vi "getEnumFromName.vi"(8 "error in (no error)":errorcluster, 10 "name":string, 11 "Enumeration in":refnum<class "Enumeration.lvclass">) -> (0 "error out":errorcluster, 3 "Enumeration out":refnum<class "Enumeration.lvclass">)   [LabVIEW 2016, in "Enumeration.lvclass"]
uses:
  Enumeration.lvclass
  Enumeration.lvclass/Enumeration.ctl
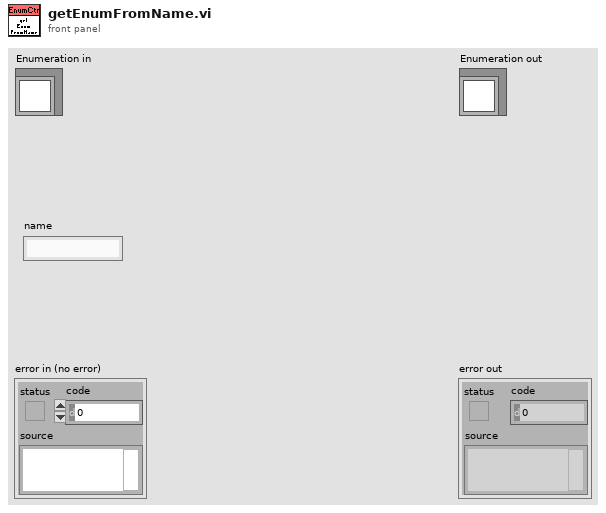
[diagram p1: front panel]
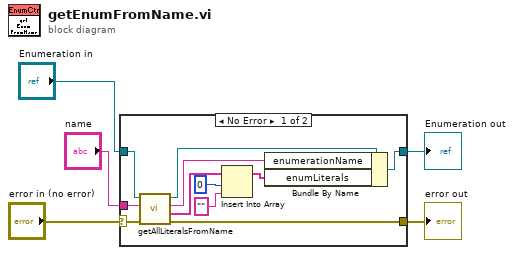
[diagram p0: block diagram]
diagram:
  n1 = case shown="No Error" "error in (no error)" {
    selector: "error in (no error)" -> [w14 w18]
    tunnel: [w7 w18] -> w4
    tunnel: [w12 w17] -> w2
    tunnel: "Enumeration in" -> [w15 w17]
    tunnel: "name" -> [w16 _]
    frame No Error {
      n2 = call "getAllLiteralsFromName.vi"("error in (no error)"=w14, "name"=w16, "Enumeration in"=w15) -> ("error out"=w7:errorcluster, "literals"=w10:string[], "name"=w11:string, "Enumeration out"=w13:refnum<class "Enumeration.lvclass">)  [unwired: 5 in]
      n3 = Insert Into Array(array=w10, index=0, new element="" ("new element/subarray")) -> (w6:string[])
      n4 = Bundle By Name(cluster=w13, "enumerationName"=w11, "enumLiterals"=w6) -> (w12:refnum<class "Enumeration.lvclass">)
    }
    frame Error {
    }
  }
  "error out" <- w4
  "Enumeration out" <- w2
